vi "SaveData.vi"(1 "Input 2D Array":string[][](array[string])) -> (0 "Success?":bool)   [LabVIEW 2016]
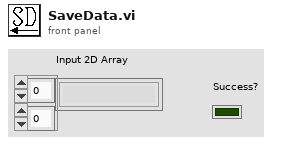
[diagram p1: front panel]
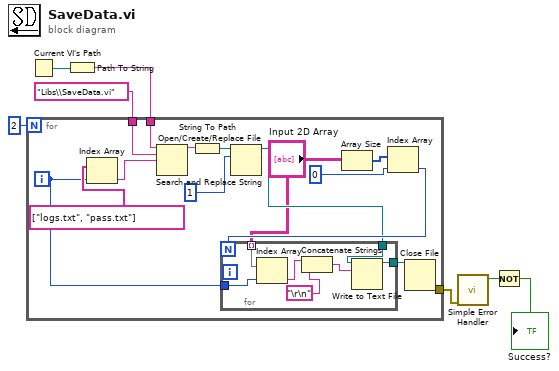
[diagram p0: block diagram]
diagram:
  n1 = Current VI's Path() -> (path=w7:path)
  n2 = Path To String(path=w7) -> (string=w5:string)
  n3 = for {
    N: 2 -> [_]
    tunnel: w5 -> [w21]
    tunnel: "Libs\\SaveData.vi" -> [w20]
    tunnel: [w8] -> w3
    i -> [w9]
    n4 = Index Array(array=string[] ["logs.txt", "pass.txt"], index=w9) -> (element=w19:string)
    n5 = Search and Replace String(input string=w21, search string=w20, replace string=w19) -> (result string=w18:string)  [unwired: 5 in, 3 out]
    n6 = String To Path(string=w18) -> (path=w17:path)
    n7 = Open/Create/Replace File(file path (use dialog)=w17, operation (0:open)=1) -> (refnum out=w13:refnum<file>)  [unwired: 4 in, 2 out]
    n8 = Array Size(array="Input 2D Array") -> (size(s)=w15:i32[])
    n9 = Index Array(array=w15, index=0) -> (element=w14:i32)
    n10 = for {
      N: w14 -> [_]
      tunnel: "Input 2D Array" -> [w29] mode=indexing
      tunnel: w13 -> [w26]
      tunnel: [w24] -> w12
      tunnel: w9 -> [w23]
      n11 = Index Array(array=w29, index=w23) -> (element=w28:string)
      n12 = Concatenate Strings(w28, "\r\n") -> (w25:string)
      n13 = Write to Text File(file (use dialog)=w26, text=w25) -> (refnum out=w24:refnum<file>)  [unwired: 2 in, 2 out]
    }
    n14 = Close File(refnum=w12) -> (error out=w8:errorcluster)  [unwired: 1 in, 1 out]
  }
  n15 = call <vilib>:"Simple Error Handler.vi"("error in (no error)"=w3) -> ("error?"=w2:bool)  [unwired: 4 in, 4 out]
  n16 = Not(x=w2) -> (.not. x?=→"Success?":bool)
